vi "SRDG535.constructor.vi"(0 "name":string, 2 "data in":string, 5 "error in":errorcluster) -> (14 "i ref out":refnum<vi>, 16 "data out":string, 19 "error out":errorcluster)   [LabVIEW 2014, in "SRDG535.lvlib"]
doc: "DG535 from Stanford Research Systems\n\nauthor: Holger Brand, PHELIX\n\nLicense Agreement for this software:\n\nCopyright (C)\nGesellschaft für Schwerionenforschung, GSI\nPlanckstr. 1\n64291 Darmstadt\nGermany\n\nContact: D.Beck@gsi.de \n\nThis program is free software; you can redistribute it and/or modify it under the terms of the \nGNU General Public License as published by the Free Software Foundation; either version 2 of \nthe license, or (at your option) any later version.\n\nThis program is distributed in the hope that it will be useful, but WITHOUT ANY WARRANTY; \nwithout even the implied warranty of MERCHANTABILITY or FITNESS FOR A PARTICULAR PURPOSE. See the GNU General License for more details (http://www.gnu.org).\n\nGesellschaft für Schwerionenforschung, GSI\nPlanckstr. 1, 64291 Darmstadt, Germany\nFor all questions and ideas contact: M.Richter@gsi.de, H.Brand@gsi.de or D.Beck@gsi.de.\nLast update: 16-JUN-2004"
uses:
  SRDG535.lvlib
  SRDG535.Delay.ctl
  SRDG535.Trigger.ctl
  CSPhelix/PH_PSDBWriter/PH_PSDBWriter.lvlib
  CSPhelix/PH_Class/PH_Class.lvlib
  CSPhelix/PH_StatusHandler/PH_StatusHandler.lvlib
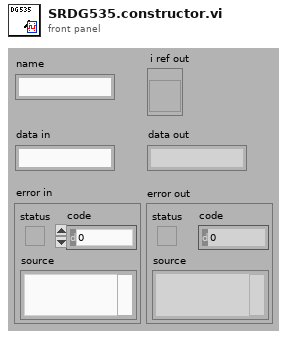
[diagram p1: front panel]
types:
  T1 = enum16{"SetAttribute", "GetAttribute", "CreateAttribute", "DestroyAttribute", "DestroyAllAtributes"}
  T2 = typedef "SRDG535.lvlib/SRDG535.Trigger.ctl" = cluster{"trigger":u32, "Impedance":bool, "Slope":bool, "burst count":i32, "external level (V)":sgl, "Internal/Burst Rate (Hz)":dbl, "Burst Period":i32}
  T3 = typedef "SRDG535.lvlib/SRDG535.Delay.ctl" = cluster{"CH A":cluster{"rel to":u32, "Delay (s)":dbl}, "CH B":cluster{"rel to":u32, "Delay (s)":dbl}, "CH C":cluster{"rel to":u32, "Delay (s)":dbl}, "CH D":cluster{"rel to":u32, "Delay (s)":dbl}}
  T4 = typedef "SRDG535.lvlib/SRDG535.i attribute.ctl" = cluster{"GPIB address":string, "Device error":errorcluster, "GUI Refs":cluster{"Delete":refnum<vi>, "Device Error":refnum<vi>, "Information":refnum<vi>, "Output":refnum<vi>, "Delay":refnum<vi>, "Trigger":refnum<vi>}, "Output Settings":T5, "Service ID Rate":i32, "Service IDs Channelinfo":i32[], "Delay Settings":T3, "Trigger Settings":T2}
  T5 = typedef "SRDG535.lvlib/SRDG535.Output.ctl" = cluster{"CH T0":T6, "CH A":T6, "CH B":T6, "CH AB":T6, "CH C":T6, "CH D":T6, "CH CD":T6}
  T6 = typedef "SRDG535.lvlib/SRDG535.Channel Output.ctl" = cluster{"Inversion":bool, "Amplitude (V)":dbl, "Offset (V)":dbl, "Mode":i32, "Load":bool}
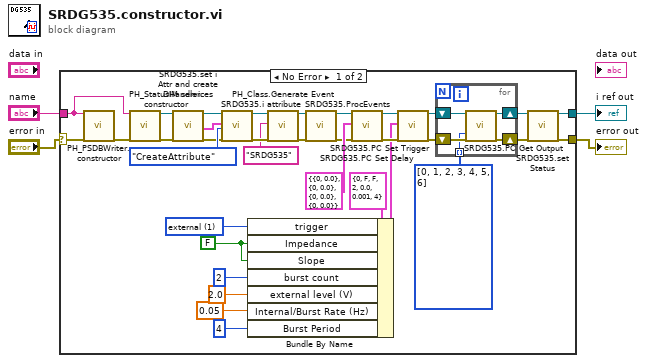
[diagram p0: block diagram]
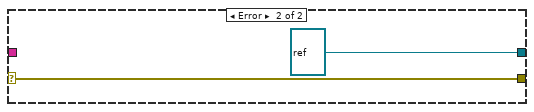
[diagram p2: hidden frame]
diagram:
  n1 = case shown="No Error" "error in" {
    selector: "error in" -> [w8 w44]
    tunnel: "name" -> [w5 _]
    tunnel: [w21 w44] -> w3
    tunnel: [w22 refnum<vi> refnum ("i ref out")] -> w2
    frame No Error {
      w36 = u16[] [0, 1, 2, 3, 4, 5, 6] items=["T0", "A", "B", "AB", "C", "D", "CD"]
      w29 = u32 1 items=["internal", "external", "single shot", "burst", "line"] ("trigger")
      w26 = FALSE ("input impedance")
      n2 = call "PH_PSDBWriter.constructor.vi"("name"=w5, "error in"=w8) -> ("error out"=w12:errorcluster)  [unwired: 15 in, 2 out]
      n3 = call "PH_StatusHandler.constructor.vi"("name"=w5, "error in(no error)"=w12) -> ("i ref out"=w6:refnum<vi>, "error out"=w7:errorcluster)  [unwired: 15 in, 1 out]
      n4 = call "SRDG535.set i Attr and create DIM services.vi"("i ref in"=w6, "error in (no error)"=w7) -> ("i ref out"=w11:refnum<vi>, "i Attributes"=w9:T4, "error out"=w10:errorcluster)  [unwired: 15 in]
      n5 = call "SRDG535.i attribute.vi"("VI Refnum"=w11, "CLASS.i attribute"=w9, "Action"=T1."CreateAttribute", "error in (no error)"=w10) -> ("VI Refnum out"=w18:refnum<vi>, "error out"=w17:errorcluster)  [unwired: 13 in, 1 out]
      n6 = Bundle By Name(cluster=T2 {"trigger"=0, "Impedance"=FALSE, "Slope"=FALSE, "burst count"=2, "external level (V)"=0.0, "Internal/Burst Rate (Hz)"=0.001, "Burst Period"=4} ("Trigger Settings"), "trigger"=w29, "Impedance"=w26, "Slope"=w26, "burst count"=2, "external level (V)"=sgl 2.0 ("external trigger level"), "Internal/Burst Rate (Hz)"=0.05 ("internal/burst trigger rate"), "Burst Period"=4 ("burst period")) -> (w23:T2)
      n7 = call "PH_Class.Generate Event.vi"("i ref in"=w18, "Class"="SRDG535", "error in (no error)"=w17) -> ("i ref out"=w19:refnum<vi>, "error out"=w20:errorcluster)  [unwired: 15 in]
      n8 = call "SRDG535.ProcEvents.vi"("i ref in"=w19, "error in"=w20) -> ("i ref out"=w14:refnum<vi>, "error out"=w13:errorcluster)  [unwired: 16 in]
      n9 = call "SRDG535.PC Set Delay.vi"("i ref in"=w14, "Delay Settings"=T3 {"CH A"={"rel to"=0, "Delay (s)"=0.0}, "CH B"={"rel to"=0, "Delay (s)"=0.0}, "CH C"={"rel to"=0, "Delay (s)"=0.0}, "CH D"={"rel to"=0, "Delay (s)"=0.0}} ("SRDG 535 Delay Settings"), "error IO"=w13) -> ("i ref out"=w35:refnum<vi>, "error out"=w33:errorcluster)  [unwired: 15 in]
      n10 = call "SRDG535.PC Set Trigger.vi"("i ref in"=w35, "Trigger Settings"=w23, "error IO"=w33) -> ("i ref out"=w34:refnum<vi>, "error out"=w32:errorcluster)  [unwired: 15 in]
      n11 = for {
        shift-right: [w43] -> w38
        shift-left: w34 -> [w42]
        shift-right: [w41] -> w37
        shift-left: w32 -> [w40]
        tunnel: w36 -> [w39] mode=indexing
        n12 = call "SRDG535.PC Get Output.vi"("i ref in"=w42, "Channel"=w39, "error IO"=w40) -> ("i ref out"=w43:refnum<vi>, "error out"=w41:errorcluster)  [unwired: 15 in]
      }
      n13 = call "SRDG535.set Status.vi"("i ref in"=w38, "error in"=w37) -> ("i ref out"=w22:refnum<vi>, "error out"=w21:errorcluster)  [unwired: 16 in]
    }
    frame Error {
    }
  }
  "i ref out" <- w2
  "error out" <- w3
